vi "Initialize SharedRsc Attribute.vi"() -> (3 "Attribute.SharedResource":refnum<class "Attribute.SharedResource.lvclass">)   [LabVIEW 2013, in "Attribute.SharedResource.lvclass"]
uses:
  Attribute.SharedResource.lvclass
  Definitions/def.SMO/Scope -- Enum.ctl
  Attribute/Attribute.lvclass/Attribute.ctl
  Attribute/Attribute.lvclass
  Definitions/def.SMO/def.SMO.lvclass
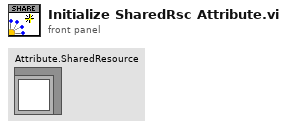
[diagram p1: front panel]
types:
  T1 = typedef "def.SMO.lvclass/Scope -- Enum.ctl" = enum16{"Public", "Protected", "Private"}
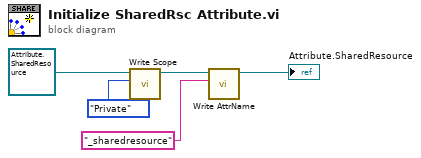
[diagram p0: block diagram]
diagram:
  n1 = call "Write Scope.vi"("Scope"=Scope_--_Enum."Private", "Attribute in"=refnum<class "Attribute.SharedResource.lvclass"> refnum ("Attribute.Owner in")) -> ("Attribute out"=w5:refnum<class "Attribute.SharedResource.lvclass">)  [unwired: 9 in]
  n2 = call "Write AttrName.vi"("Attribute Name"="_sharedresource", "Attribute in"=w5) -> ("Attribute out"=→"Attribute.SharedResource":refnum<class "Attribute.SharedResource.lvclass">)  [unwired: 9 in]
